vi "Read Program Control Event.vi"(8 "error in (no error)":errorcluster, 11 "Universal Robot in":refnum<class "Universal Robot.lvclass">) -> (0 "error out":errorcluster, 2 "Program Control Event":refnum<user-event>, 3 "Universal Robot out":refnum<class "Universal Robot.lvclass">)   [LabVIEW 2019, in "Universal Robot.lvclass"]
uses:
  Universal Robot.lvclass
  ProgramControlEvent.ctl
  Universal Robot.lvclass/Universal Robot.ctl
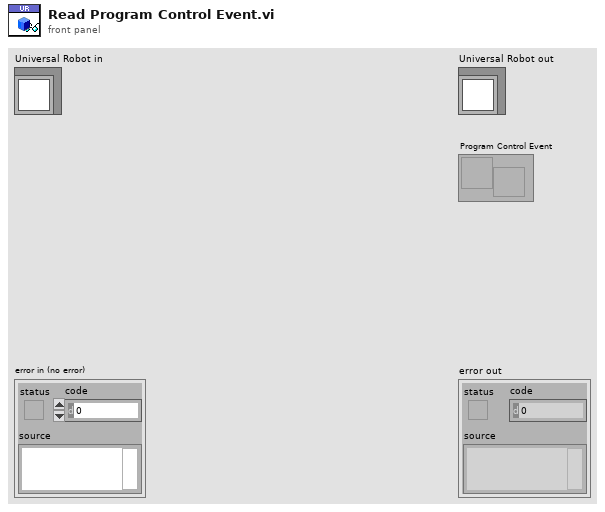
[diagram p1: front panel]
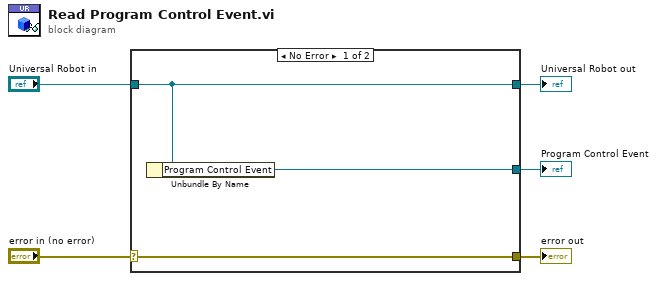
[diagram p0: block diagram]
diagram:
  n1 = case shown="No Error" "error in (no error)" {
    selector: "error in (no error)" -> [w8 w9]
    tunnel: [w8 w9] -> w4
    tunnel: [w7 w10] -> w2
    tunnel: "Universal Robot in" -> [w7 w10]
    tunnel: [w6 _] -> w1
    frame No Error {
      n2 = Unbundle By Name(w7) -> ("Program Control Event"=w6:refnum<user-event>)
    }
    frame Error {
    }
  }
  "error out" <- w4
  "Universal Robot out" <- w2
  "Program Control Event" <- w1
